vi "Init.vi"(8 "error in (no error)":errorcluster, 10 "Resource":refnum<class "DeployResource.lvclass">, 11 "Platform":refnum<class "DeployPlatform.lvclass">) -> (0 "error out":errorcluster, 3 "Device out":refnum<class "Device.lvclass">)   [LabVIEW 2020, in "PicoG-App.lvlib" / "Device.lvclass"]
uses:
  Device.lvclass
  Builds/picoG/ppl/PicoG-Core.lvlibp/PicoG-Processor/PicoG-Core/DeployPlatform/DeployPlatform.lvclass
  Builds/picoG/ppl/PicoG-Core.lvlibp/PicoG-Processor/PicoG-Core/DeployResource/DeployResource.lvclass
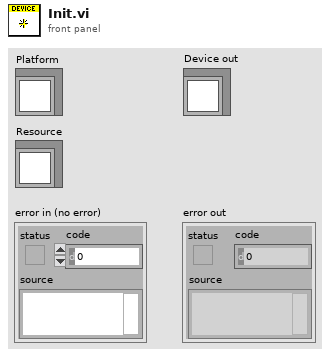
[diagram p1: front panel]
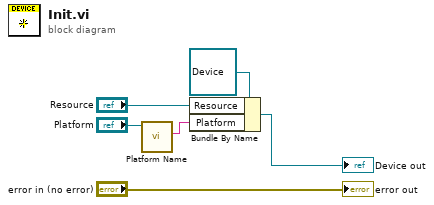
[diagram p0: block diagram]
diagram:
  n1 = call-dynamic "Platform Name.vi"("DeployTarget in"="Platform") -> ("Platform Name"=w2:string)  [unwired: 8 in, 2 out]
  n2 = Bundle By Name(cluster=refnum<class "Device.lvclass"> refnum ("Device in"), "Resource"="Resource", "Platform"=w2) -> (→"Device out":refnum<class "Device.lvclass">)
  "error out" <- "error in (no error)"
